vi "Point-Truncating.vi"() -> ()   [LabVIEW 2014]
panel:
  out "Result":dbl
  in  "truncate digit places":i32
  in  "Number":dbl
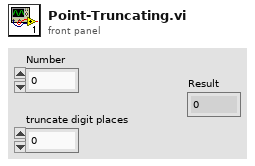
[diagram p1: front panel]
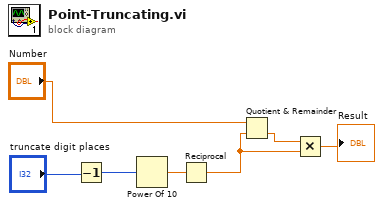
[diagram p0: block diagram]
diagram:
  n1 = Decrement(x="truncate digit places") -> (x-1=w6:i32)
  n2 = Power Of 10(x=w6) -> (10^x=w5:dbl)
  n3 = Reciprocal(x=w5) -> (1/x=w2:dbl)
  n4 = Quotient & Remainder(x="Number", y=w2) -> (floor(x/y)=w3:dbl)  [unwired: 1 out]
  n5 = Multiply(x=w3, y=w2) -> (x*y=→"Result":dbl)
